vi "Different Sinks for Multiple Loggers Example.vi"() -> ()   [LabVIEW 2020]
uses:
  Source/Type Defs/Debug Level.ctl
  Source/Sinks/File Sink/File Sink.lvclass
  C:/Users/hughe_cx/Documents/05_repos/LVLog/Source/Sinks/Sink/Sink.lvclass
  Source/LV Log.lvlib
  Source/Logger/Logger.lvclass
panel:
  in  "Log Path 2":path
  in  "Log Path":path
  in  "error in (no error)":errorcluster
  out "error out":errorcluster
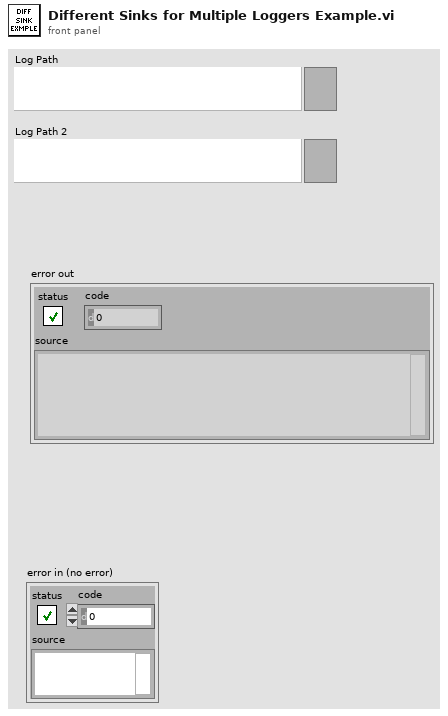
[diagram p1: front panel]
types:
  T1 = typedef "LV Log.lvlib/Debug Level.ctl" = enum16{"DEFAULT", "DEBUG", "INFO", "WARN", "ERROR", "FATAL"}
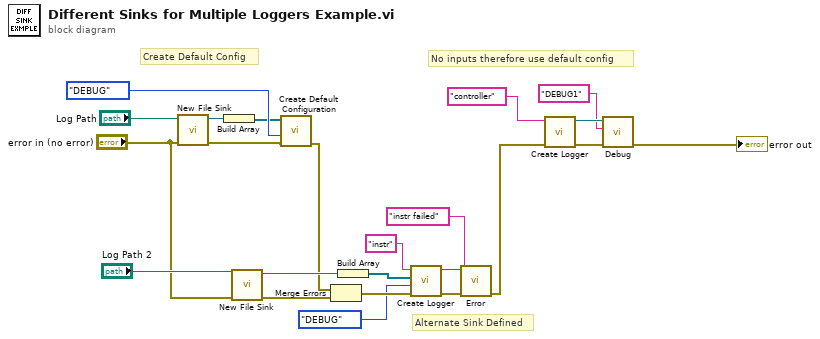
[diagram p0: block diagram]
diagram:
  # "Alternate Sink Defined"
  # "No inputs therefore use default config"
  # "Create Default Config"
  n1 = call "New File Sink.vi"("error in (no error)"="error in (no error)", "File Path"="Log Path") -> ("error out"=w4:errorcluster, "File Sink out"=w2:refnum<class "File Sink.lvclass">)  [unwired: 8 in]
  n2 = Build Array(w2) -> (w1:refnum<class "File Sink.lvclass">[])
  n3 = call "New File Sink.vi"("error in (no error)"="error in (no error)", "File Path"="Log Path 2") -> ("error out"=w12:errorcluster, "File Sink out"=w11:refnum<class "File Sink.lvclass">)  [unwired: 8 in]
  n4 = call "Create Default Configuration.vi"("Sinks"=w1, "Debug Level in"=Debug_Level."DEBUG" ("Debug Level"), "error in (no error)"=w4) -> ("error out"=w5:errorcluster)  [unwired: 7 in]
  n5 = Merge Errors(w5, w12) -> (w13:errorcluster)
  n6 = Build Array(w11) -> (w10:refnum<class "File Sink.lvclass">[])
  n7 = call "Create Logger.vi"("error in (no error)"=w13, "Debug Level (Default)"=Debug_Level."DEBUG" ("Debug Level in"), "Sinks (Default)"=w10, "Name"="instr") -> ("error out"=w15:errorcluster, "Logger out"=w16:refnum<class "Logger.lvclass">)  [unwired: 6 in]
  n8 = call "Error.vi"("error in (no error)"=w15, "Log Text"="instr failed", "Logger in"=w16) -> ("error out"=w17:errorcluster)  [unwired: 6 in, 2 out]
  n9 = call "Create Logger.vi"("error in (no error)"=w17, "Name"="controller") -> ("error out"=w22:errorcluster, "Logger out"=w21:refnum<class "Logger.lvclass">)  [unwired: 8 in]
  n10 = call "Debug.vi"("error in (no error)"=w22, "Log Text"="DEBUG1", "Logger in"=w21) -> ("error out"=→"error out":errorcluster)  [unwired: 6 in, 2 out]
